vi "GT Get Axis Config.vi"(8 "error in (no error)":errorcluster caption="错误输入（无错误）", 9 "pAxis":T1, 10 "axis":i16, 11 "cardNum":i16) -> (0 "error out":errorcluster caption="错误输出", 1 "pAxis out":T1, 3 "function return":i16)   [LabVIEW 2020, in "gts1.lvlib"]
doc: "GT_API GT_GetAxisConfig(short cardNum,short axis,TAxisConfig *pAxis);"
uses:
  gts1.lvlib
  dll/32bit/multi_card/gts.dll
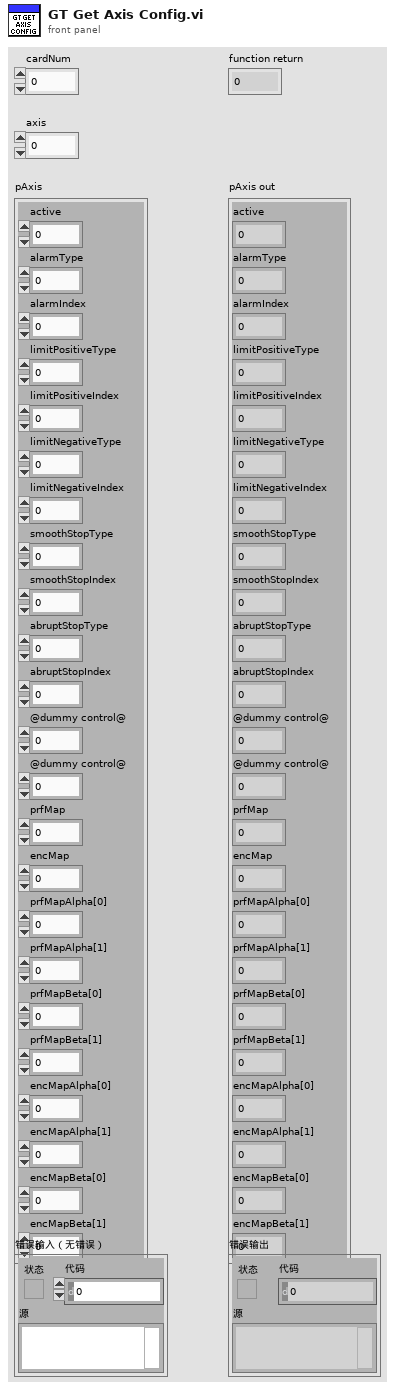
[diagram p1: front panel]
types:
  T1 = cluster{"active":i16, "alarmType":i16, "alarmIndex":i16, "limitPositiveType":i16, "limitPositiveIndex":i16, "limitNegativeType":i16, "limitNegativeIndex":i16, "smoothStopType":i16, "smoothStopIndex":i16, "abruptStopType":i16, "abruptStopIndex":i16, "@dummy control@":i8, "@dummy control@":i8, "prfMap":i32, "encMap":i32, "prfMapAlpha[0]":i16, "prfMapAlpha[1]":i16, "prfMapBeta[0]":i16, "prfMapBeta[1]":i16, "encMapAlpha[0]":i16, "encMapAlpha[1]":i16, "encMapBeta[0]":i16, "encMapBeta[1]":i16}
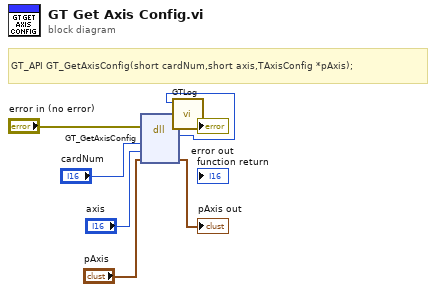
[diagram p0: block diagram]
diagram:
  # "GT_API GT_GetAxisConfig(short cardNum,short axis,TAxisConfig *pAxis);"
  n1 = dll-call lib="C:/1228/dll/32bit/multi_card/gts.dll" fn="GT_GetAxisConfig"(error in="error in (no error)", "cardNum"="cardNum", "axis"="axis", "pAxis"="pAxis") -> (error out=w3:errorcluster, w1:i16, "pAxis"=→"pAxis out":T1)  [unwired: 4 in, 1 out]
  n2 = call "GTLog.vi"("error in (no error)"=w3, "Numeric"=w1) -> ("error out"=→"error out":errorcluster)  [unwired: 9 in]
